vi "gaussian.vi"() -> ()   [LabVIEW 2018]
uses:
  <vilib>/Utility/file.llb/Read Delimited Spreadsheet (DBL).vi
  <vilib>/gmath/statdist.llb/Normal CDF.vi
  <vilib>/gmath/NI_Gmath.lvlib
panel:
  out "Prepared by \nthe project":string
  out "Gaussian Probabilty Function":dbl(graph)
  out "Data":dbl[][](array[numeric])
  in  "Measurement file \nwith extension Txt":path
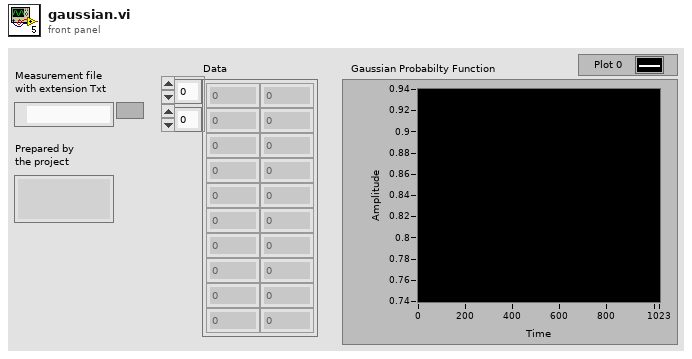
[diagram p1: front panel]
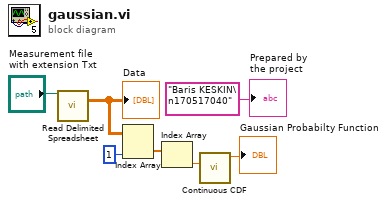
[diagram p0: block diagram]
diagram:
  n1 = call-poly <vilib>:"Read Delimited Spreadsheet.vi"("file path (dialog if empty)"="Measurement file \nwith extension Txt") -> ("all rows"=w6:dbl[][])  [unwired: 9 in, 5 out]
  "Data" <- w6
  n2 = Index Array(array=w6, index (col)=1 ("disabled index (col)")) -> (element=w5:dbl[])  [unwired: 1 in]
  n3 = Index Array(array=w5) -> (element=w3:dbl)  [unwired: 1 in]
  n4 = call-poly <vilib>:"Continuous CDF.vi"("x"=w3) -> ("cdf(x)"=→"Gaussian Probabilty Function":dbl)  [unwired: 9 in, 1 out]
  "Prepared by \nthe project" <- "Baris KESKIN\n170517040"
